vi "SDSU_MultAttHandling.vi"(8 "error IO":errorcluster, 10 "arguments":string, 11 "refnum":i32) -> (0 "err out":errorcluster, 2 "response":string, 3 "refnum out":i32)   [LabVIEW 2016]
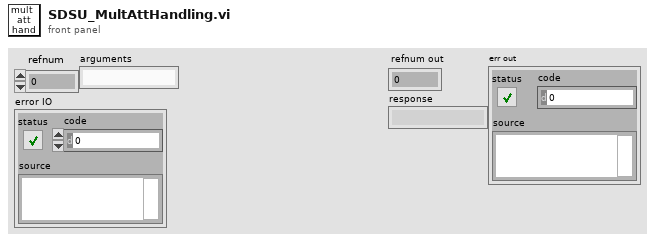
[diagram p1: front panel]
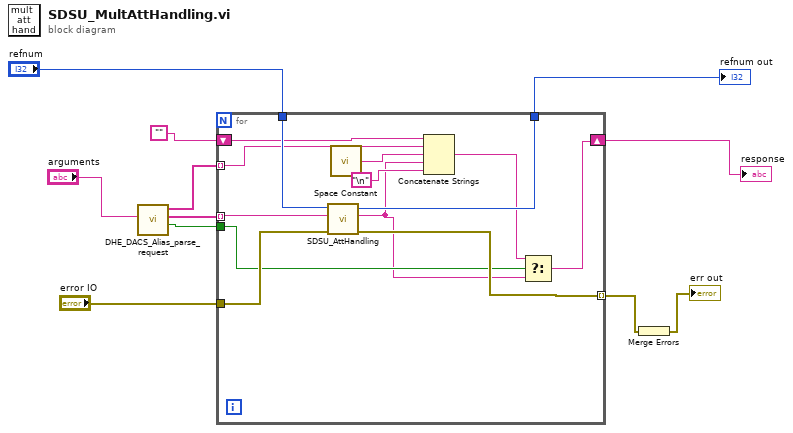
[diagram p0: block diagram]
diagram:
  n1 = call "DHE_DACS_Alias_parse_request.vi"("cmd in"="arguments") -> ("mult. aliases?"=w4:bool, "cmds out"=w8:string[], "alias names"=w6:string[])  [unwired: 7 in, 1 out]
  n2 = for {
    tunnel: "refnum" -> [w24]
    tunnel: [w23] -> w9
    tunnel: w8 -> [w22] mode=indexing
    tunnel: "error IO" -> [w21]
    tunnel: [w20] -> w2 mode=indexing
    tunnel: w6 -> [w18] mode=indexing
    shift-right: [w12] -> w3
    shift-left: "" -> [w19]
    tunnel: w4 -> [w15]
    n3 = call "SDSU_AttHandling.vi"("error IO"=w21, "arguments"=w22, "refnum"=w24) -> ("err out"=w20:errorcluster, "response"=w14:string, "refnum out"=w23:i32)  [unwired: 6 in]
    n4 = call <vilib>:"Space Constant.vi"() -> ("String"=w17:string)
    n5 = Concatenate Strings(w19, w18, w17, w14, "\n") -> (w13:string)
    n6 = Select(t=w13, s=w15, f=w14) -> (s? t:f=w12:string)
  }
  "refnum out" <- w9
  "response" <- w3
  n7 = Merge Errors(w2) -> (→"err out":errorcluster)
